vi "Init Actor Core.vi"(8 "error in (no error)":errorcluster, 11 "App in":refnum<class "App.lvclass">) -> (0 "error out":errorcluster, 3 "App out":refnum<class "App.lvclass">)   [LabVIEW 2016, in "App.lvlib" / "App.lvclass"]
uses:
  App.lvclass
  App.lvclass/App.ctl
  Dynamic Instrument/Dynamic Instrument/Dynamic Instrument.lvclass
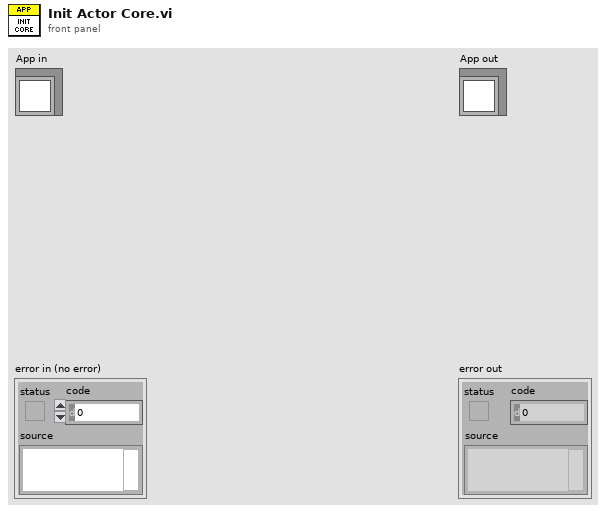
[diagram p1: front panel]
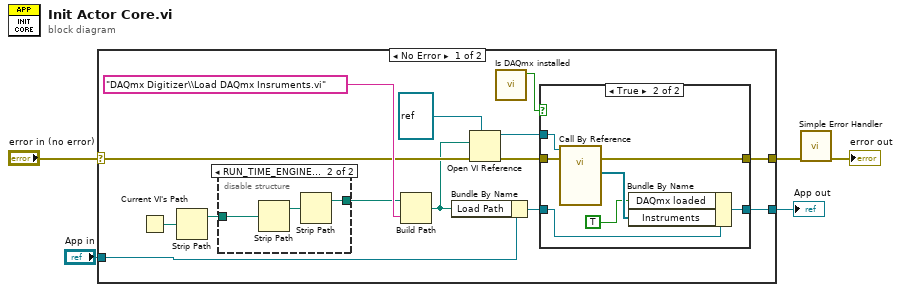
[diagram p0: block diagram]
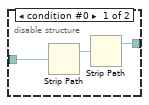
[diagram p2: hidden frame]
diagram:
  n1 = case shown="No Error" "error in (no error)" {
    selector: "error in (no error)" -> [w11 w36]
    tunnel: [w10 w36] -> w4
    tunnel: [w12 w35] -> w2
    tunnel: "App in" -> [w13 w35]
    frame No Error {
      n2 = Current VI's Path() -> (path=w17:path)
      n3 = Strip Path(path=w17) -> (stripped path=w9:path)  [unwired: 1 out]
      n4 = disable-structure shown="RUN_TIME_ENGINE==False" {
        disable-tunnel: w9 -> [w22 w23]
        disable-tunnel: [w20 w25] -> w8
        frame condition #0 {
          n5 = Strip Path(path=w22) -> (stripped path=w21:path)  [unwired: 1 out]
          n6 = Strip Path(path=w21) -> (stripped path=w20:path)  [unwired: 1 out]
        }
        frame condition #1 (active) {
          n7 = Strip Path(path=w23) -> (stripped path=w24:path)  [unwired: 1 out]
          n8 = Strip Path(path=w24) -> (stripped path=w25:path)  [unwired: 1 out]
        }
      }
      n9 = Build Path(base path=w8, name or relative path="DAQmx Digitizer\\Load DAQmx Insruments.vi") -> (appended path=w6:path)
      n10 = Bundle By Name(cluster=w13, "Load Path"=w6) -> (w7:refnum<class "App.lvclass">)
      n11 = Open VI Reference(type specifier VI Refnum (for type only)=refnum<vi> refnum, vi path=w6, error in (no error)=w11) -> (vi reference=w15:refnum<vi>, error out=w14:errorcluster)  [unwired: 3 in]
      n12 = call "Is DAQmx installed.vi"() -> ("file or folder exists?"=w19:bool)  [unwired: 11 in]
      n13 = case shown="True" w19 {
        tunnel: w15 -> [_ w34]
        tunnel: w14 -> [w26 w33]
        tunnel: w7 -> [w27 w32]
        tunnel: [w27 w31] -> w12
        tunnel: [w26 w28] -> w10
        frame False {
        }
        frame True {
          n14 = call-by-ref "?"(reference=w34, error in=w33) -> (error out=w28:errorcluster, "Instruments"=w30:refnum<class "Dynamic Instrument.lvclass">[])  [unwired: 11 in, 1 out]
          n15 = Bundle By Name(cluster=w32, "DAQmx loaded"=TRUE, "Instruments"=w30) -> (w31:refnum<class "App.lvclass">)
        }
      }
    }
    frame Error {
    }
  }
  "App out" <- w2
  n16 = call <vilib>:"Simple Error Handler.vi"("error in (no error)"=w4) -> ("error out"=→"error out":errorcluster)  [unwired: 4 in, 4 out]
